vi "Configure Averaging.vi"(7 "Enable Averaging (T: Enable)":bool=TRUE, 8 "error in (no error)":errorcluster, 9 "Averaging Type (0: Auto)":i32(ring) items=["Auto", "RMS", "Log", "Scalar"], 10 "Average Count (100)":i32=100, 11 "VISA resource name":refnum<visa-resource-name>) -> (0 "error out":errorcluster, 3 "VISA resource name out":refnum<visa-resource-name>)   [LabVIEW 2018, in "Agilent MXA Series.lvlib"]
doc: "Configures the averaging.\n\n<B>Note:</B>\nYou can use this VI only under Burst Power and Swept SA measurement types."
uses:
  Agilent MXA Series.lvlib
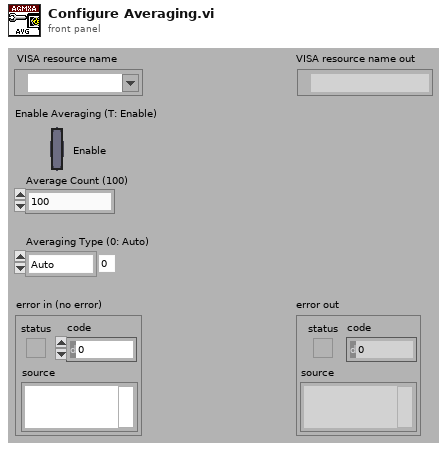
[diagram p1: front panel]
types:
  T1 = typedef "Agilent MXA Series.lvlib/Extended User Data.ctl" = cluster{"Measurement Type":i32, "Agilent MXA/EXA Model":i32}
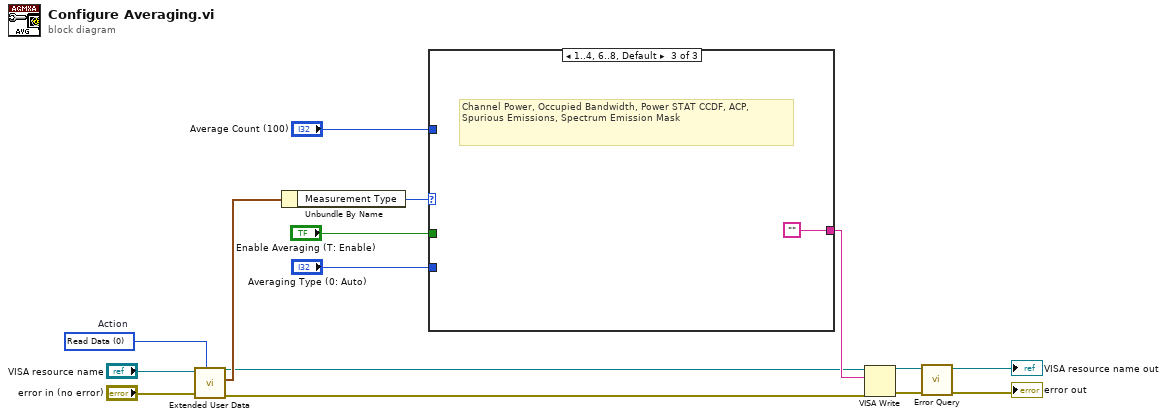
[diagram p0: block diagram]
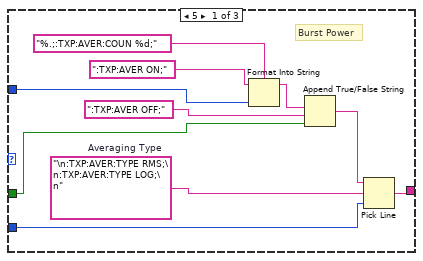
[diagram p2: hidden frame]
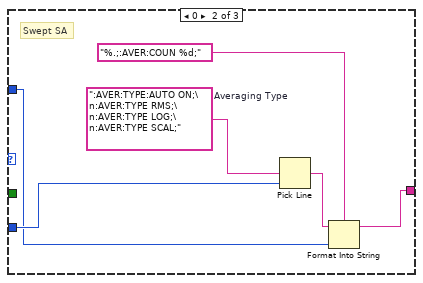
[diagram p3: hidden frame]
diagram:
  w7 = 0 items=["Read Data", "Write Data", "Clear Data", "Clear ALL Data"]  # Action
  n1 = call "Extended User Data.vi"("Action (1:Write Data)"=w7, "Error In (no error)"="error in (no error)", "VISA resource name in"="VISA resource name") -> ("Error Out"=w9:errorcluster, "User Data Out"=w6:T1, "VISA resource name out"=w1:refnum<visa-resource-name>)  [unwired: 6 in]
  n2 = Unbundle By Name(w6) -> ("Measurement Type"=w5:i32)
  n3 = case shown="1..4, 6..8, Default" w5 {
    tunnel: [w20 w28 ""] -> w15
    tunnel: "Averaging Type (0: Auto)" -> [w23 w27 _]
    tunnel: "Average Count (100)" -> [w22 w26 _]
    tunnel: "Enable Averaging (T: Enable)" -> [w21 _ _]
    frame 5 {
      w25 = "\n:TXP:AVER:TYPE RMS;\n:TXP:AVER:TYPE LOG;\n"  # Averaging Type
      # "Burst Power"
      n4 = Format Into String(format string="%.;:TXP:AVER:COUN %d;", initial string=":TXP:AVER ON;" ("false string"), w22) -> (resulting string=w16:string)  [unwired: 1 in, 1 out]
      n5 = Append True/False String(1:w21, 2:":TXP:AVER OFF;" ("false string"), 3:w16) -> (0:w17:string)  [unwired: 1 in]
      n6 = Pick Line(string ("")=w17, multi-line string=w25, line index=w23) -> (output string=w20:string)
    }
    frame 0 {
      w31 = ":AVER:TYPE:AUTO ON;\n:AVER:TYPE RMS;\n:AVER:TYPE LOG;\n:AVER:TYPE SCAL;"  # Averaging Type
      # "Swept SA"
      n7 = Pick Line(multi-line string=w31, line index=w27) -> (output string=w29:string)  [unwired: 1 in]
      n8 = Format Into String(format string="%.;:AVER:COUN %d;", initial string=w29, w26) -> (resulting string=w28:string)  [unwired: 1 in, 1 out]
    }
    frame 1..4, 6..8, Default {
      # "Channel Power, Occupied Bandwidth, Power STAT CCDF, ACP,\nSpurious Emissions, Spectrum Emission Mask"
    }
  }
  n9 = VISA Write(VISA resource name=w1, write buffer=w15, error in (no error)=w9) -> (VISA resource name out=w13:refnum<visa-resource-name>, error out=w14:errorcluster)  [unwired: 1 out]
  n10 = call "Error Query.vi"("error in (no error)"=w14, "VISA resource name"=w13) -> ("error out"=→"error out":errorcluster, "VISA resource name out"=→"VISA resource name out":refnum<visa-resource-name>)  [unwired: 6 in, 2 out]
